vi "TRACTION WRITE FGV.vi"(7 "Enum - Menu":T1, 8 "error in (no error)":errorcluster, 11 "main ref":T2) -> (0 "error out":errorcluster)   [LabVIEW 2025]
uses:
  controls/LAB-IQ UI Data.ctl
  Traction Receipe Enum.ctl
  Traction Write enum.ctl
  d526d67c-090a-4194-9932-463c49b325c5.vi
panel:
  out "connection ID":refnum<k16>
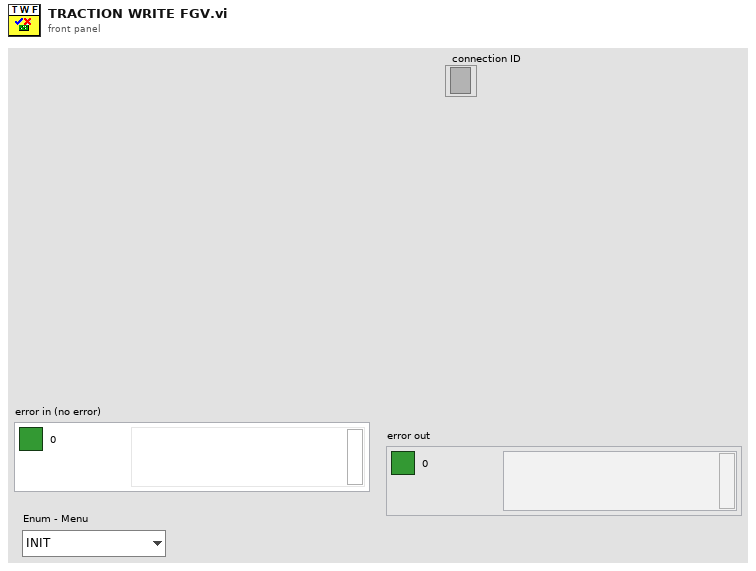
[diagram p1: front panel]
types:
  T1 = typedef "Traction Write enum.ctl" = enum16{"INIT", "WRITE", "CLOSE", "REINIT"}
  T2 = typedef "LAB-IQ UI Data.ctl" = cluster{"Main Home Screen":cluster{"GUI":refnum<vi>, "Platform Settings":refnum<vi>, "Configure":refnum<vi>, "Home":refnum<vi>, "EXIT":refnum<vi>, "service 2":refnum<vi>, "MainPage":refnum<vi>, "Analysis":refnum<vi>}, "Platform Settings":cluster{"mm/s  Surge":refnum<vi>, "Update Surge Speed":refnum<vi>, "Drive Error":refnum<vi>, "Disable Axis Jog Soft Limits":refnum<vi>, "mm/s  Sway":refnum<vi>, "Sway and Surge COM Status":refnum<vi>, "Heave COM Status":refnum<vi>, "Enable Platform":refnum<vi>, "Surge Forward Main":refnum<vi>, "Sway Right Main":refnum<vi>, "Sway Left Main":refnum<vi>, "Heave Down Main":refnum<vi>, "Heave Up main":refnum<vi>, "Update Sway Speed":refnum<vi>, "Update Heave Speed":refnum<vi>, "mm/s Heave":refnum<vi>, "mm/sec":refnum<vi>, "mm":refnum<vi>, "Surge Backward Main":refnum<vi>}, "Analysis Screen":cluster{"Analysis Home":refnum<vi>, "Surface Analysis":refnum<vi>, "Imaging":refnum<vi>, "Image Analysis":refnum<vi>, "Post Analysis":refnum<vi>}, "Config Screen":cluster{"Select Load Head":refnum<vi>, "Notes :":refnum<vi>, "FILE":refnum<vi>, "Sample ID :":refnum<vi>, "Operator ID :":refnum<vi>, "Operator Name :":refnum<vi>, "Auto":refnum<vi>}, "Motion Module":cluster{"zNL":refnum<vi>, "NL disp":refnum<vi>, "Rotary Tab":refnum<vi>, "Motion Direction:  3":refnum<vi>, "E.Velocity 2":refnum<vi>, "e.v/ssr 2":refnum<vi>, "Enter Fixed E.Velocity 2":refnum<vi>, "Enter Final SRR 2":refnum<vi>, "Enter initial SRR 2":refnum<vi>, "Enter Fixed SRR 2":refnum<vi>, "Enter the Final E.Velocity (m/s) 2":refnum<vi>, "Enter initial E.Velocity (m/s) 2":refnum<vi>, "Final Speed (RPM) 3":refnum<vi>, "Initial Speed (RPM) 2":refnum<vi>, "Enter the Final Velocity (m/s) 3":refnum<vi>, "Enter initial Velocity (m/s)  3":refnum<vi>, "Ramp Up 2":refnum<vi>, "TEST SELECTION":refnum<vi>, "SPEED SELECTION : ":refnum<vi>, "Angular Oscillation Set":refnum<vi>, "Traction":refnum<vi>, "Step Speed":refnum<vi>, "StepTable For Load-Speed":refnum<vi>, "StepTable For Speed":refnum<vi>, "Surge Forward MM":refnum<vi>, "Surge Backward MM":refnum<vi>, "M3 Image":refnum<vi>, "String 39":refnum<vi>, "Sway Left MM":refnum<vi>, "Sway Right MM":refnum<vi>, "Disable Axis Jog Soft Limits":refnum<vi>, "mm":refnum<vi>, "Heave Down MM":refnum<vi>, "Heave Up MM":refnum<vi>, "Wear Track Diameter (mm)":refnum<vi>, "Set WTD":refnum<vi>, "HomeScratch":refnum<vi>, "HomeRot":refnum<vi>, "PlaceModule":refnum<vi>, "Enter the Angle (Deg)":refnum<vi>, "Enter the Frequency (Hz)":refnum<vi>, "Motion Mode:":refnum<vi>, "LR Sway":refnum<vi>, "Rot Hor":refnum<vi>, "Scratch":refnum<vi>, "LR Cam":refnum<vi>, "MMBack":refnum<vi>, "MMNext":refnum<vi>, "Rot Ver":refnum<vi>, "Rotary Module Selection":refnum<vi>, "calculate rotary":refnum<vi>, "SPEED SELECTION : rotary":refnum<vi>, "Import 2":refnum<vi>, "Save 2":refnum<vi>, "File Path :  2":refnum<vi>, "String 45":refnum<vi>, "StepTable For Speed 3":refnum<vi>, "Enter the Speed(mm/sec)":refnum<vi>, "Enter the Speed(RPM)":refnum<vi>, "Enter Scratch Speed (mm/s):":refnum<vi>, "SwaySpeed Set":refnum<vi>, "Scartch Offset":refnum<vi>, "Motion type:":refnum<vi>, "HomeScratch 2":refnum<vi>, "Enter Scratch length (mm):":refnum<vi>, "Wear Track Diameter":refnum<vi>, "Rotary Speed Exced":refnum<vi>, "Scratch Mode":refnum<vi>, "No of Scratch":refnum<vi>}, "Environmental control":cluster{"Humidity  Status  3":refnum<vi>, "Low Temp  Status  2":refnum<vi>, "TK4 status 2":refnum<vi>, "Stage Temperature":refnum<vi>, "Sample Temperature":refnum<vi>, "Humidity (Amb)":refnum<vi>, "Clear List":refnum<vi>, "Add to list":refnum<vi>, "Wear":refnum<vi>, "Vibration":refnum<vi>, "Humidity (Chamber)":refnum<vi>, "Temperature (Chamber)":refnum<vi>, "ECR ":refnum<vi>, "Temperature (Amb)":refnum<vi>, "Microphone":refnum<vi>, "Acoustic Emission 3":refnum<vi>, "SNext":refnum<vi>, "APBack":refnum<vi>, "Enter the Temperature (°C):":refnum<vi>, "Enter the Stage \nTemperature (°C):":refnum<vi>, "Enter the Humidity (%Rh):":refnum<vi>, "Low Temp":refnum<vi>, "High Temp":refnum<vi>, "Humidity":refnum<vi>, "Sensors Picked":refnum<vi>}, "About Screen":cluster{"Password":refnum<vi>, "Home Service":refnum<vi>, "Advanced Setting":refnum<vi>, "About Tab":refnum<vi>, "ECR Port:":refnum<vi>, "Ramp Port:":refnum<vi>, "Installation/Replacement completed":refnum<vi>, "Loahead":refnum<vi>, "Heave and Surge COM Port:":refnum<vi>, "Sway COM Port:":refnum<vi>, "Temp Modbus:":refnum<vi>, "Humidity Port:":refnum<vi>, "Edit Gain Constants":refnum<vi>, "Save Gain Constants":refnum<vi>}, "Main Screen":cluster{"Main Screen Tab":refnum<vi>, "Angle and Frequency":refnum<vi>, "Stroke (mm)":refnum<vi>, "Angle (Deg)":refnum<vi>, "Main Speed Tab":refnum<vi>, "MTM MOTOR DISPLAY":refnum<vi>, "Disc Speed (m/sec)":refnum<vi>, "Ball Speed (m/sec)":refnum<vi>, "Disc Speed (RPM)":refnum<vi>, "Ball Speed (RPM)":refnum<vi>, "SPEED TAB":refnum<vi>, "Speed (m/sec)":refnum<vi>, "Set Speed (m/sec)":refnum<vi>, "Speed (RPM)":refnum<vi>, "Set Speed":refnum<vi>, "Time Tab":refnum<vi>, "Time ( HH:MM:SS ) 2":refnum<vi>, "Test Duration":refnum<vi>, "Test Duration 4":refnum<vi>, "TEST CYCLE":refnum<vi>, "TOTAL CYCLES":refnum<vi>, "Set Load (N)":refnum<vi>, "Temp Tabs":refnum<vi>, "Heater":refnum<vi>, "TK4 status":refnum<vi>, "ChamberTemp":refnum<vi>, "SetTmp":refnum<vi>, "Controller  Status":refnum<vi>, "ChamberTemp 2":refnum<vi>, "SetTmp 2":refnum<vi>, "Controller  Status 2":refnum<vi>, "ChamberTemp 3":refnum<vi>, "SetTmp 3":refnum<vi>, "Cooling":refnum<vi>, "Load Communication":refnum<vi>, "Ambient \nTemperature":refnum<vi>, "HumCOMStatus":refnum<vi>, "Ambient\n Humidity":refnum<vi>, "Freq (Hz)":refnum<vi>, "Load En":refnum<vi>, "NLt":refnum<vi>, "zNL 2":refnum<vi>, "Humidity On":refnum<vi>, "humidity disp":refnum<vi>, "Set Humidity":refnum<vi>, "NL disp 2":refnum<vi>, "Humidity On 2":refnum<vi>, "humidity disp 2":refnum<vi>, "Set Humidity 2":refnum<vi>, "NL disp 3":refnum<vi>, "AppLoadSeq scratch":refnum<vi>, "Stop Scratch":refnum<vi>, "ClrLog":refnum<vi>, "Trip Log":refnum<vi>, "STOP":refnum<vi>, "Start Test":refnum<vi>, "Test status":refnum<vi>, "AR Led":refnum<vi>, "Data":refnum<vi>, "Health":refnum<vi>, "Sway COM Status":refnum<vi>, "Heave COM Status":refnum<vi>, "Grp Tab":refnum<vi>, "Sub Graph":refnum<vi>, "SD (mm)":refnum<vi>, "Siliding distance Reset Graph":refnum<vi>, "SDGp":refnum<vi>, "Humidity Reset Graph":refnum<vi>, "HumrGp":refnum<vi>, "Acoustic Emission (mV)":refnum<vi>, "Aqucostic Reset Graph":refnum<vi>, "gACQUOS":refnum<vi>, "ECR RESET":refnum<vi>, "ECR":refnum<vi>, "Temperature Reset":refnum<vi>, "Acoustic Emission (mV) 2":refnum<vi>, "Aqucostic Reset Graph 2":refnum<vi>, "gACQUOS 2":refnum<vi>, "ECR RESET 2":refnum<vi>, "ECR 2":refnum<vi>, "Temperature Reset 2":refnum<vi>, "Temperature (deg c)":refnum<vi>, "Speed Reset Graph":refnum<vi>, "Speed Tab":refnum<vi>, "MTM DISC  SPEED":refnum<vi>, "MTM BALL SPEED":refnum<vi>, "speed mm/sec":refnum<vi>, "Hymidity":refnum<vi>, "Humidity Disable trip":refnum<vi>, "CoF Trip  2":refnum<vi>, "Depth Trip":refnum<vi>, "Weart Deapth":refnum<vi>, "Depth Reset Graph":refnum<vi>, "Weart":refnum<vi>, "Depthz":refnum<vi>, "Depth (µm)":refnum<vi>, "WearGp":refnum<vi>, "NL Trip 2":refnum<vi>, "Load pid":refnum<vi>, "Load Disable Trip":refnum<vi>, "Load Reset Graph":refnum<vi>, "NL Display 4":refnum<vi>, "Main Chart 3":refnum<vi>, "BACK":refnum<vi>, "Depth Trip 2":refnum<vi>, "COF TRIP ":refnum<vi>, "Friction Force (N)":refnum<vi>, "FF Reset Graph":refnum<vi>, "FF Disable Trip":refnum<vi>, "FF TRIP":refnum<vi>, "COF Disable Trip":refnum<vi>, "COF Reset Graph":refnum<vi>, "Start Test Temp":refnum<vi>, "zFF":refnum<vi>, "Friction Force (N) Graph":refnum<vi>, "Coefficient of Friction":refnum<vi>, "Scratch Start Test":refnum<vi>, "FF Tab":refnum<vi>, "Cyclic Friction Force (N)":refnum<vi>, "CZ FF":refnum<vi>, "Cyclic Friction Force (N) Graph":refnum<vi>, "Cyclic Coefficient of Friction":refnum<vi>, "Cyclic FF TRIP":refnum<vi>, "Cyclic FF Disable Trip":refnum<vi>, "cyclic COF Disable Trip":refnum<vi>, "cyclic COF TRIP":refnum<vi>, "cyclic COF Reset Graph":refnum<vi>, "Cyclic FF Reset Graph":refnum<vi>, "Test Trip":refnum<vi>, "Multi Scratch Pass":refnum<vi>, "Scratch Start Recording":refnum<vi>}, "Loading":cluster{"Indentation":refnum<vi>, "Reference Sample":refnum<vi>, "Load Cell Communication Slide":refnum<vi>, "com 3":refnum<vi>, "com":refnum<vi>, "DecaForce COM Status":refnum<vi>, "Update":refnum<vi>, "Clear 3":refnum<vi>, "seq":refnum<vi>, "Stribeck table":refnum<vi>, "Stribeck Table  For loading":refnum<vi>, "Loading Mode":refnum<vi>, "Enter the Final Load (N)":refnum<vi>, "Enter the CoF Trip":refnum<vi>, "Enter the Friction Force Trip":refnum<vi>, "Enter the Normal load Trip":refnum<vi>, "Enter the Load  (N)":refnum<vi>, "KiloForce":refnum<vi>, "DecaForce ":refnum<vi>, "MicroForce":refnum<vi>, "LHBack":refnum<vi>, "LHNext":refnum<vi>, "Enter the Loading Rate (N/min)":refnum<vi>, "Message":refnum<vi>, "Warning 2":refnum<vi>, "SSP 0.75":refnum<vi>, "SSP 0.5":refnum<vi>, "SSP 0.3":refnum<vi>, "Warning":refnum<vi>, "gui GIF":refnum<vi>, "Communication is established":refnum<vi>, "AppLoad 4":refnum<vi>, "Multipoint":refnum<vi>, "Load Selection":refnum<vi>}, "PID":cluster{"Ramp MulFac":refnum<vi>, "pulses LoadDiffRamp(2..10)":refnum<vi>, "PulseControlRamp(diff<=3N)":refnum<vi>, "SetLoadDeadband(%) Load(0-10N)":refnum<vi>, "PID gains out delay (microForce)":refnum<vi>, "Ramp":refnum<vi>, "Gain 2":refnum<vi>, "pulses LoadDiff(2..10)":refnum<vi>, "pulses LoadDiff(11..50)":refnum<vi>, "PulseControl(diff<=3N)":refnum<vi>, "SetLoadDeadband(%)  2":refnum<vi>, "Dummy Run":refnum<vi>, "Vertical load (N)":refnum<vi>, "AutoTune":refnum<vi>, "Offset 3 ":refnum<vi>, "apply load":refnum<vi>, "Offset  3":refnum<vi>, "apply load 2":refnum<vi>, "Enter ByPass Load":refnum<vi>, "reinit 3":refnum<vi>, "output range delay":refnum<vi>, "PID gains out delay":refnum<vi>, "Bypass Load":refnum<vi>, "pulsesSent":refnum<vi>, "pulses ":refnum<vi>, "actpid":refnum<vi>, "gFF Rot":refnum<vi>, "pulses LoadDiff(21..1000)":refnum<vi>, "Delay":refnum<vi>, "deadband":refnum<vi>}, "Config Parameters":cluster{"Tab Control 3":refnum<vi>, "Tab Control 19":refnum<vi>, "SAMPLES":refnum<vi>, "Re-initilaize":refnum<vi>, "Filter ON/OFF":refnum<vi>, "TracHomeSurgeOffsetCounts 10MM":refnum<vi>, "TracHomeSwayOffsetCounts 10MM":refnum<vi>, "Acoustic Emission:":refnum<vi>, "Apply Filter (FF)":refnum<vi>, "Filter% 2":refnum<vi>, "Apply Filter (Load)":refnum<vi>, "Filter% ":refnum<vi>, "Sway distance (mm)":refnum<vi>, "Surge distance (mm)":refnum<vi>, "DataSavingLoopDelay(ms)":refnum<vi>, "SAVE 2":refnum<vi>, "Enter Distance":refnum<vi>, "Sway Counts:":refnum<vi>, "Distance (mm): 3":refnum<vi>, "Surge Counts:":refnum<vi>, "Distance (mm): 2":refnum<vi>, "Distance (mm):":refnum<vi>, "Heave Counts:":refnum<vi>, "LRMHomeSurgeOffsetCounts":refnum<vi>, "LRMHomeSwayOffsetCounts":refnum<vi>, "TracHomeSurgeOffsetCounts 20MM":refnum<vi>, "TracHomeSwayOffsetCounts 20MM":refnum<vi>, "RotHomeSwayOffsetCounts":refnum<vi>, "RotHomeSurgeOffsetCounts":refnum<vi>, "Heave distance":refnum<vi>, "Zmm":refnum<vi>, "Heave Pulses/mm":refnum<vi>, "Surge Pulses/mm":refnum<vi>, "Sway Pulses/mm":refnum<vi>, "Heave Pitch":refnum<vi>, "Surge Pitch":refnum<vi>, "Sway Pitch":refnum<vi>, "Heave PPR":refnum<vi>, "Surge PPR":refnum<vi>, "Sway PPR":refnum<vi>, "Tab Control 5":refnum<vi>, "Tab Control 14":refnum<vi>, "Tab Control 26":refnum<vi>, "AE":refnum<vi>, "Heave Loop Delay":refnum<vi>, "Heave PID Speed":refnum<vi>, "Surge Jog Speed":refnum<vi>, "Heave Jog Speed":refnum<vi>, "Sway Loop Delay":refnum<vi>, "Sway PID Speed":refnum<vi>, "Sway Jog Speed":refnum<vi>, "DEPTH TRIP VALUE":refnum<vi>, "LOAD TRIP VALUE":refnum<vi>, "DEPTH TRIP   ENABLE":refnum<vi>, "LOAD TRIP  ENABLE":refnum<vi>, "CYCLIC FF TRIP VALUE":refnum<vi>, "FF TRIP VALUE":refnum<vi>, "CYCLIC CoF TRIP VALUE":refnum<vi>, "COF TRIP VALUE":refnum<vi>, "CYCLIC COF TRIP  ENABLE":refnum<vi>, "CYCLIC FF TRIP  ENABLE":refnum<vi>, "FF TRIP  ENABLE":refnum<vi>, "COF TRIP  ENABLE":refnum<vi>, "JOG TRIP LOAD VALUE (N)":refnum<vi>}, "Loading Com Port":cluster{"ClearAll":refnum<vi>, "Mz(Nm)":refnum<vi>, "My(Nm)":refnum<vi>, "Mx(Nm)":refnum<vi>, "Save Dwell":refnum<vi>, "Mx ":refnum<vi>, "My ":refnum<vi>, "Mz":refnum<vi>, "Fx(N)":refnum<vi>, "Fy(N)":refnum<vi>, "Fz(N)":refnum<vi>, "ZeroAll":refnum<vi>, "Acq Delay (ms)":refnum<vi>, "Burst Delay (ms)":refnum<vi>, "model":refnum<vi>, "SN":refnum<vi>, "FFx(N)":refnum<vi>, "Sensor IP":refnum<vi>, "Port":refnum<vi>, "FFy(N)":refnum<vi>, "Load(N)":refnum<vi>, "delete Handle":refnum<vi>, "Create Handle":refnum<vi>, "ft_data":refnum<vi>, "ft_range":refnum<vi>, "ft_data 2":refnum<vi>, "stop 6":refnum<vi>, "running_flag":refnum<vi>, "ft_udp_handle":refnum<vi>, "get-data-return":refnum<vi>, "get-range-return":refnum<vi>, "zero-return":refnum<vi>, "filter-return":refnum<vi>, "initial-return":refnum<vi>, "deleteHandle-result":refnum<vi>, "Load Cell Temp":refnum<vi>}, "Heave AND Surge":cluster{"SURGE POSE":refnum<vi>, "error out Read":refnum<vi>, "HEAVE POSE":refnum<vi>, "State":refnum<vi>, "Homed":refnum<vi>, "Sequence ID":refnum<vi>, "error out Write":refnum<vi>, "faultCode":refnum<vi>, "Ack ID":refnum<vi>, "SPEED":refnum<vi>, "Distance":refnum<vi>, "Mode Command":refnum<vi>, "Heave and Surge Read":refnum<vi>, "Read Heave Temp":refnum<vi>, "Spare 15":refnum<vi>, "Spare 14":refnum<vi>, "Spare 13":refnum<vi>, "Spare 12":refnum<vi>, "Spare 11":refnum<vi>, "Spare 10":refnum<vi>, "Spare 9":refnum<vi>, "Spare 8":refnum<vi>, "Spare 7":refnum<vi>, "Spare 6":refnum<vi>, "Spare 5":refnum<vi>, "Spare 4":refnum<vi>, "Spare 2":refnum<vi>, "Spare 1":refnum<vi>, "Node Id":refnum<vi>, "Spare 3":refnum<vi>, "SPARE 4":refnum<vi>, "SPARE 3":refnum<vi>, "SPARE 2":refnum<vi>, "SPARE 1":refnum<vi>, "fwMajor":refnum<vi>, "fwMinor":refnum<vi>, "Manual Write":refnum<vi>, "Heave and Surge Write":refnum<vi>, "SPARE 5":refnum<vi>, "Reserved ":refnum<vi>, "SPARE 8":refnum<vi>, "SPARE 6":refnum<vi>, "SPARE 7":refnum<vi>, "SPARE 17":refnum<vi>, "SPARE 16":refnum<vi>, "SPARE 15":refnum<vi>, "SPARE 14":refnum<vi>, "SPARE 13":refnum<vi>, "SPARE 12":refnum<vi>, "SPARE 11":refnum<vi>, "SPARE 10":refnum<vi>, "SPARE 9":refnum<vi>, "System UPTIME":refnum<vi>, "Missed Packets":refnum<vi>, "faultCode Surge Right":refnum<vi>, "faultCode Surge Left":refnum<vi>, "faultCode Heave":refnum<vi>}, "New PID LOGIC":cluster{"Fine Tune Zone":refnum<vi>, "PID SDelay":refnum<vi>, "Max_pos_limit":refnum<vi>, "Min_pos_limit":refnum<vi>, "i_limit":refnum<vi>, "pct_scale":refnum<vi>, "Deadband":refnum<vi>, "Kd":refnum<vi>, "Ki":refnum<vi>, "Kp":refnum<vi>, "Current Position":refnum<vi>, "Set Load":refnum<vi>, "Current Load":refnum<vi>, "Pulse delta":refnum<vi>, "Init Step":refnum<vi>, "Max Step Linit":refnum<vi>, "min_deadband_floor":refnum<vi>, "dynamic_spindle_noise_scalar":refnum<vi>, "min_finetune_floor":refnum<vi>, "filter_alpha":refnum<vi>}, "SWAY ":cluster{"fwMajor":refnum<vi>, "Homed":refnum<vi>, "Rotary POSE":refnum<vi>, "State":refnum<vi>, "SWAY POSE":refnum<vi>, "Ack ID":refnum<vi>, "faultCode":refnum<vi>, "Node Id":refnum<vi>, "fwMinor":refnum<vi>, "Spare 6":refnum<vi>, "Spare 5":refnum<vi>, "Spare 4":refnum<vi>, "Spare 3":refnum<vi>, "Spare 2":refnum<vi>, "Spare 1":refnum<vi>, "Spare 7":refnum<vi>, "SPARE  5":refnum<vi>, "error out Write  SWAY ":refnum<vi>, "error out Read SWAY ":refnum<vi>, "Manual Write SWAY ":refnum<vi>, "SWAY WRITE":refnum<vi>, "SPARE  4":refnum<vi>, "SPARE  3":refnum<vi>, "SPARE 2":refnum<vi>, "SPARE 1":refnum<vi>, "Spare 15":refnum<vi>, "Spare 14":refnum<vi>, "Spare 13":refnum<vi>, "Spare 12":refnum<vi>, "Spare 11":refnum<vi>, "Spare 9":refnum<vi>, "Spare 8":refnum<vi>, "SPEED":refnum<vi>, "Distance":refnum<vi>, "Mode Command":refnum<vi>, "Sequence ID":refnum<vi>, "SWAY READ":refnum<vi>, "Spare 10":refnum<vi>, "Read SWAY Temp":refnum<vi>, "faultCode Sway ":refnum<vi>, "Missed Packets":refnum<vi>, "System UPTIME sway":refnum<vi>, "SPARE 6":refnum<vi>, "SPARE 7":refnum<vi>, "SPARE 9":refnum<vi>, "SPARE 11":refnum<vi>, "SPARE 10":refnum<vi>, "SPARE 8":refnum<vi>, "SPARE 13":refnum<vi>, "SPARE 12":refnum<vi>, "SPARE 17":refnum<vi>, "SPARE 16":refnum<vi>, "SPARE 15":refnum<vi>, "SPARE 14":refnum<vi>, "Reserved":refnum<vi>, "faultCode Rotary":refnum<vi>}, "Analysis Screen":cluster{"Analysis Home":refnum<vi>, "Refresh 2":refnum<vi>, "MEAN 4":refnum<vi>, "SD 4":refnum<vi>, "VARIANCE 4":refnum<vi>, "MEAN  3":refnum<vi>, "SD  3":refnum<vi>, "VARIANCE  3":refnum<vi>, "MEAN 2":refnum<vi>, "SD  2":refnum<vi>, "VARIANCE 2":refnum<vi>, "MEAN":refnum<vi>, "SD":refnum<vi>, "VARIANCE":refnum<vi>, "File 4 Discription":refnum<vi>, "OPEN 4":refnum<vi>, "File Name 4":refnum<vi>, "OPEN 3":refnum<vi>, "File 3 Discription":refnum<vi>, "File Name 3":refnum<vi>, "Y-AXIS":refnum<vi>, "X-AXIS":refnum<vi>, "XY Graph":refnum<vi>, "File Name 2":refnum<vi>, "File Name 1":refnum<vi>, "OPEN 2":refnum<vi>, "OPEN 1":refnum<vi>, "File 1 Discription ":refnum<vi>, "File 2 Discription":refnum<vi>, "Export":refnum<vi>, "File Format":refnum<vi>}, "Traction":cluster{"faultCode Traction 2":refnum<vi>, "faultCode Traction 1":refnum<vi>, "Missed Packets":refnum<vi>, "System UPTIME Traction":refnum<vi>, "SPARE 17":refnum<vi>, "SPARE 16":refnum<vi>, "SPARE 15":refnum<vi>, "SPARE 14":refnum<vi>, "SPARE 13":refnum<vi>, "SPARE 12":refnum<vi>, "SPARE 11":refnum<vi>, "SPARE 10":refnum<vi>, "SPARE 9":refnum<vi>, "SPARE 8":refnum<vi>, "SPARE 7":refnum<vi>, "SPARE 6":refnum<vi>, "Reserved":refnum<vi>, "SPARE  5":refnum<vi>, "Manual Write TRACTION":refnum<vi>, "TRACTION WRITE":refnum<vi>, "SPARE  4":refnum<vi>, "SPARE  3":refnum<vi>, "SPARE 2":refnum<vi>, "SPARE 1":refnum<vi>, "Spare 7":refnum<vi>, "Spare 6":refnum<vi>, "Spare 5":refnum<vi>, "Spare 4":refnum<vi>, "Spare 2":refnum<vi>, "Spare 1":refnum<vi>, "Node Id":refnum<vi>, "Read TRACTION Temp":refnum<vi>, "fwMinor":refnum<vi>, "fwMajor":refnum<vi>, "faultCode":refnum<vi>, "TRACTION POSE":refnum<vi>, "TRACTION POSE 2":refnum<vi>, "Homed":refnum<vi>, "State":refnum<vi>, "Ack ID":refnum<vi>, "SPEED":refnum<vi>, "Distance":refnum<vi>, "Mode Command":refnum<vi>, "Sequence ID":refnum<vi>, "error out Read TRACTION":refnum<vi>, "error out Write  TRACTION":refnum<vi>, "TRACTION READ":refnum<vi>, "Spare 3":refnum<vi>}, "Traction reciepe":cluster{"SRR Sweep Range (%) Stribeck":refnum<vi>, "Traction Receipe":refnum<vi>, "Total Execution Time":refnum<vi>, "Total Steps":refnum<vi>, "Duration / Step (s)  Stribeck":refnum<vi>, "STRIBECK Fixed SRR List (%)":refnum<vi>, "Duration / Step (s) Traction":refnum<vi>, "SRR Sweep Range (%) traction":refnum<vi>, "Rolling Speed (mm/s)":refnum<vi>, "Temperature Stages (°C)":refnum<vi>, "Ball Load (N)":refnum<vi>, "Lubricant Name":refnum<vi>, "Profile File Name":refnum<vi>, "SET entrainment Velocity":refnum<vi>, "Test Array Size":refnum<vi>, "SRR INDEX [ STRIBECK]":refnum<vi>, "Stribeck Size":refnum<vi>, "SET SRR":refnum<vi>, "ELAPSED TIMER ":refnum<vi>, "BALL SET RPM":refnum<vi>, "DISC SET RPM":refnum<vi>, "SET LOAD":refnum<vi>, "TEMPERATURE READ":refnum<vi>, "SET TEMPERATURE":refnum<vi>, "Traction Size":refnum<vi>, "DISC SPEED (rpm)":refnum<vi>, "BALL SPEED (rpm)":refnum<vi>, "BALL WEAR TRACK":refnum<vi>, "DISC WEARTRACK":refnum<vi>, "SRR INDEX [ TRACTION]":refnum<vi>, "Start Index Type":refnum<vi>, "Enum - Menu":refnum<vi>, "Ball (mm/sec)":refnum<vi>, "Disc (mm/sec)":refnum<vi>}, "Traction Control":cluster{"HomeTraction":refnum<vi>, "Demo Mode Display":refnum<vi>, "Traction Message":refnum<vi>, "Traction Step Update Details":refnum<vi>, "Main Tab sequence for selection":refnum<vi>, "Ramp Tab":refnum<vi>, "e.v/ssr":refnum<vi>, "Enter Fixed E.Velocity":refnum<vi>, "Enter Final SRR":refnum<vi>, "Enter initial SRR":refnum<vi>, "Enter Fixed SRR":refnum<vi>, "Enter the Final E.Velocity (m/s)":refnum<vi>, "Enter initial E.Velocity (m/s)":refnum<vi>, "Ball WTD":refnum<vi>, "E.Velocity":refnum<vi>, "Enter the Final Velocity (m/s)":refnum<vi>, "Enter initial Velocity (m/s)":refnum<vi>, "Ramp Up   Disc":refnum<vi>, "Initial DiscSpeed (RPM)":refnum<vi>, "Final Speed (RPM) Ball":refnum<vi>, "Final Speed (RPM)":refnum<vi>, "Initial Speed (RPM) Ball":refnum<vi>, "Enter the Final Velocity (m/s) Ball":refnum<vi>, "Enter initial Velocity (m/s) Ball":refnum<vi>, "Ramp Up":refnum<vi>, "ExceedBallSpeed step":refnum<vi>, "ExceedDiscSpeed":refnum<vi>, "BallSpeed Exceed Indication":refnum<vi>, "Apply":refnum<vi>, "SPEED SELECTION : MTM":refnum<vi>, "SPEED SELECTION : MTM 2":refnum<vi>, "TEST SELECTION (MTM)":refnum<vi>, "MTM Test Selection":refnum<vi>, "File Path Tab":refnum<vi>, "File Path String":refnum<vi>, "Save":refnum<vi>, "Save  2":refnum<vi>, "Import ":refnum<vi>, "File Path :":refnum<vi>, "Step Sequence Indication Tab":refnum<vi>, "Step Sequence Indication":refnum<vi>, "Calculate Step":refnum<vi>, "StepTable":refnum<vi>, "ExceedDiscSpeed  Cinstant Speed":refnum<vi>, "ExceedBallSpeed Constant":refnum<vi>, "TEST SELECTION (MTM) 2":refnum<vi>, "SPEED SELECTION : MTM 3":refnum<vi>, "MTM Test Selection 2":refnum<vi>, "Enter the Speed (m/sec): ":refnum<vi>, "Enter the Speed (m/sec):  2":refnum<vi>, "Enter the Speed (RPM):":refnum<vi>, "Lower Spped ":refnum<vi>, "Upper":refnum<vi>, "Enter the Speed (RPM):Ball":refnum<vi>, "Disc Motion Direction: ":refnum<vi>, "Ball Motion Direction :":refnum<vi>, "Motion Mode: ":refnum<vi>, "Wear Track Diameter (mm) ":refnum<vi>, "Disc Speed Indicator":refnum<vi>, "ExceedBallSpeed":refnum<vi>}}
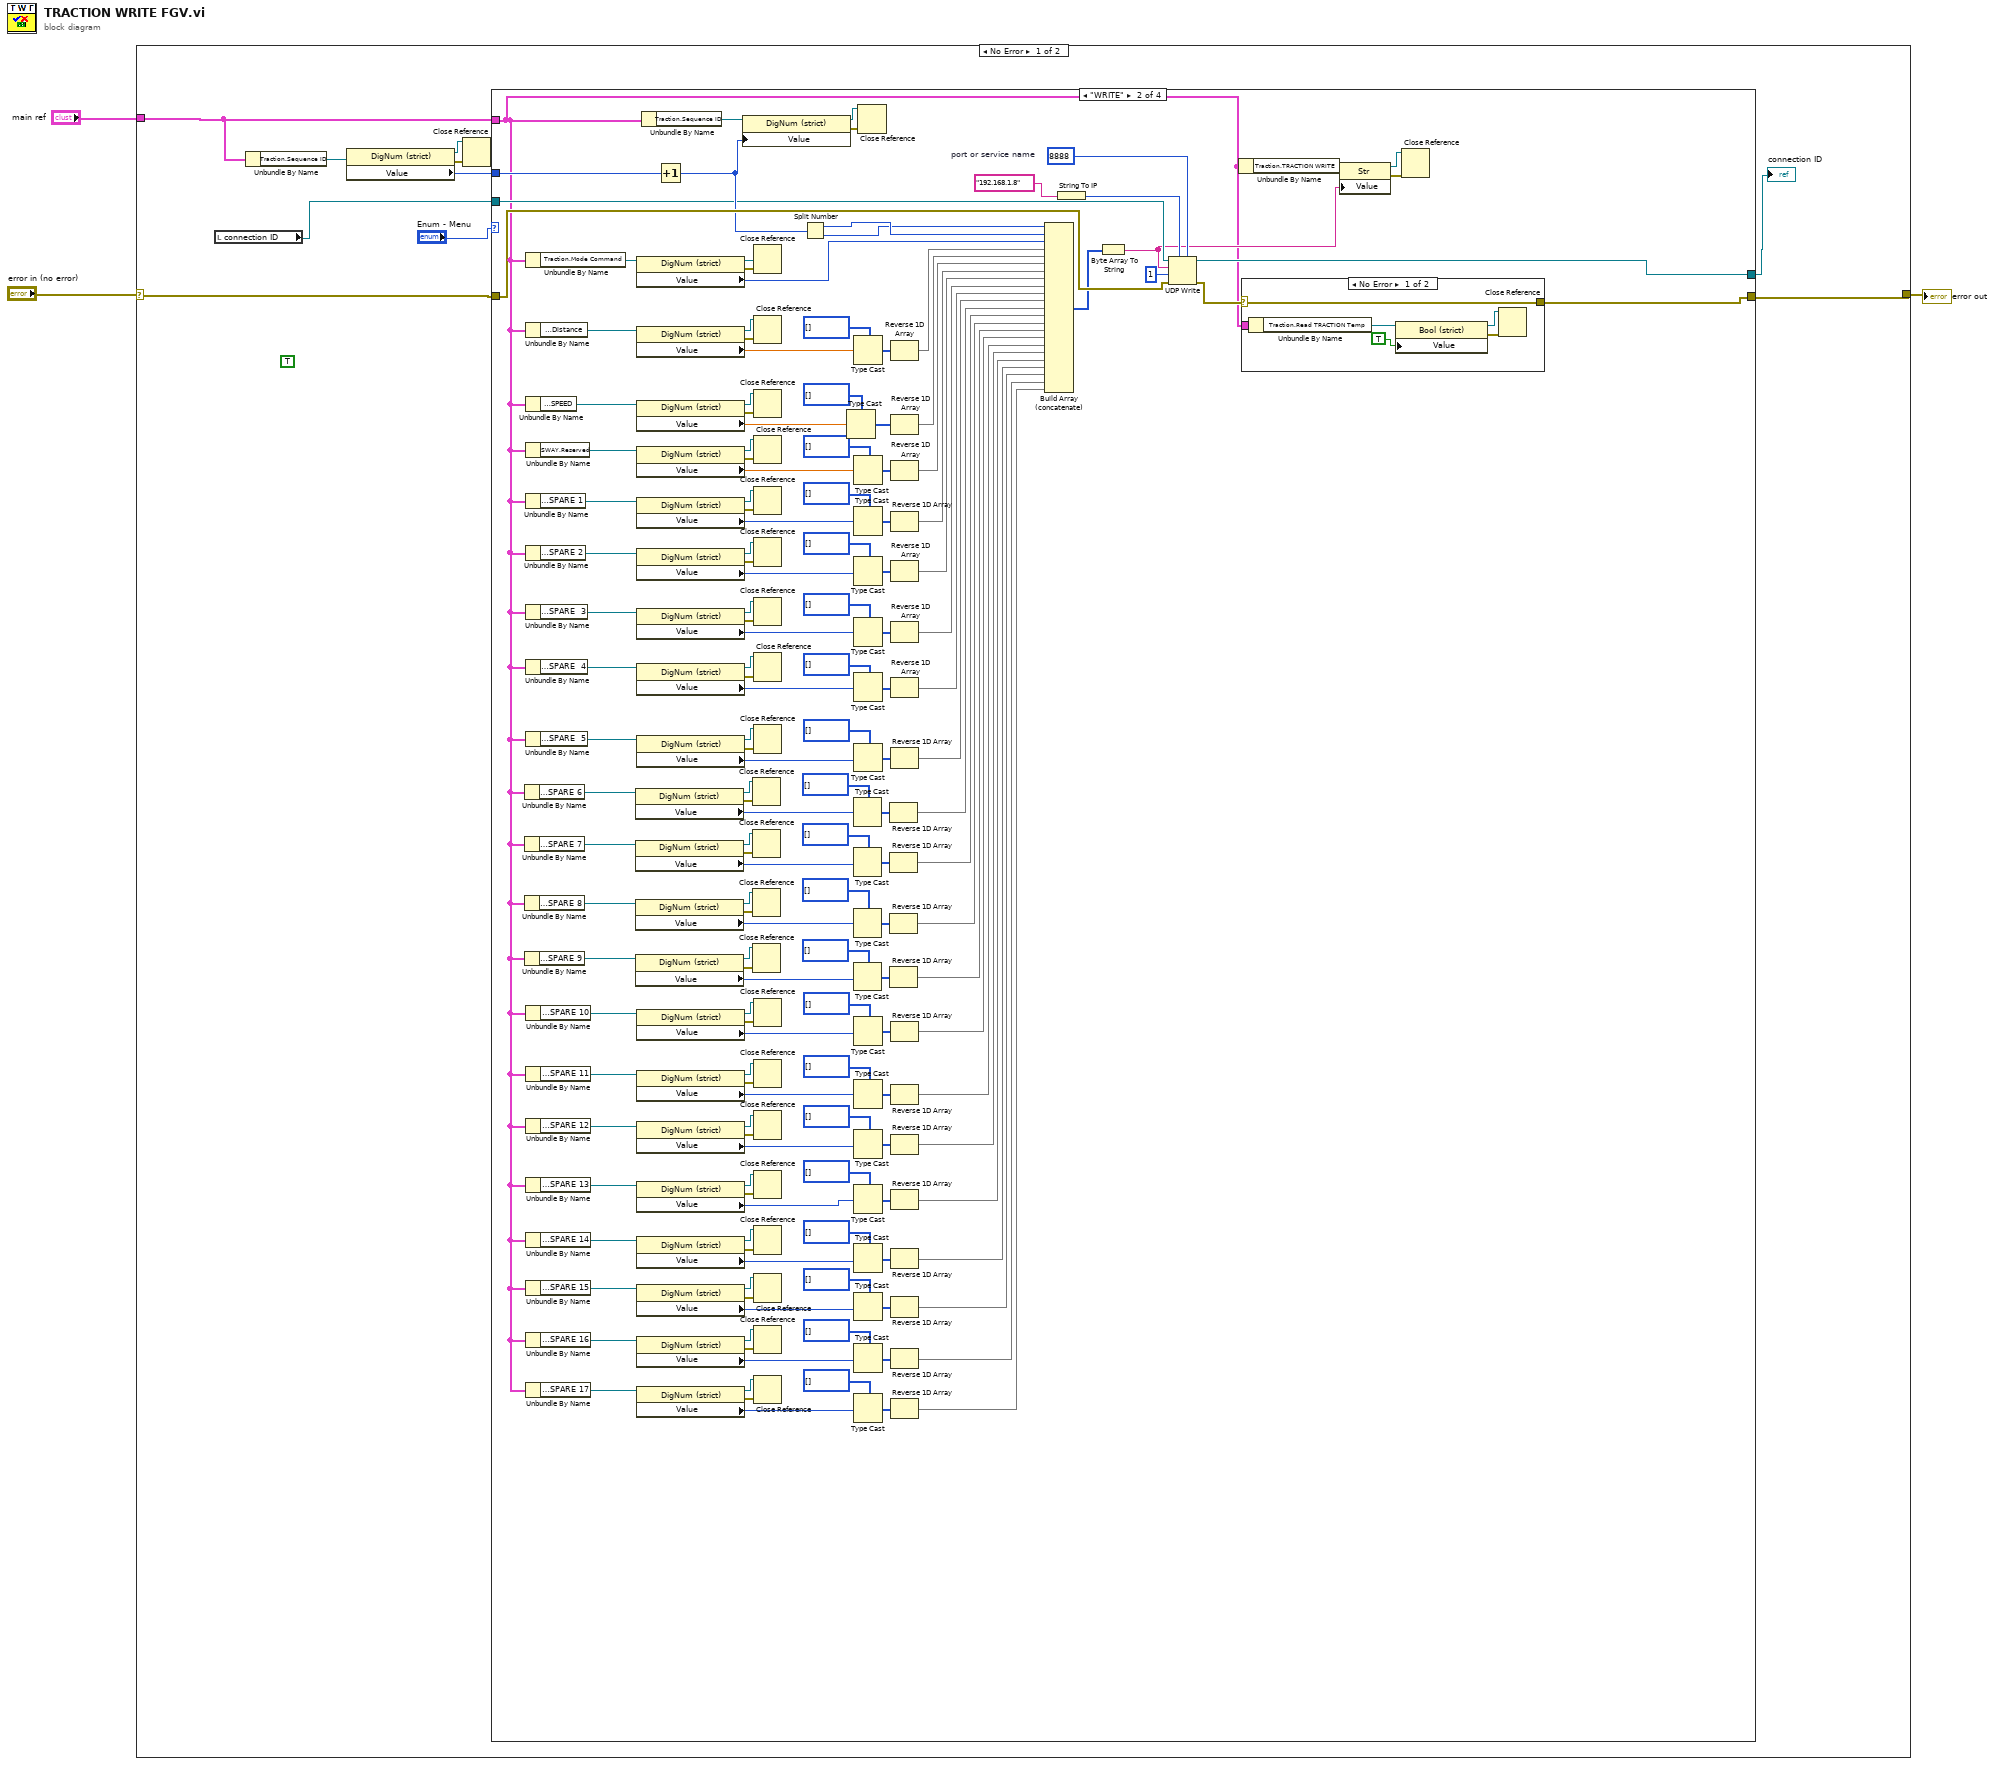
[diagram p0: block diagram]
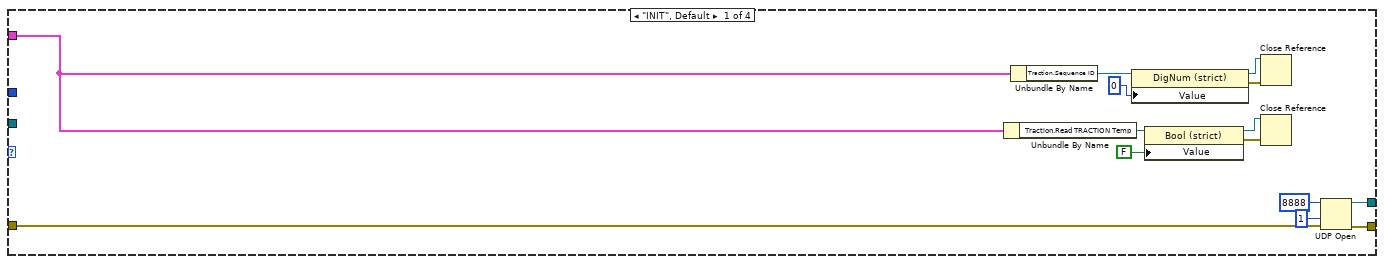
[diagram p2: hidden frame]
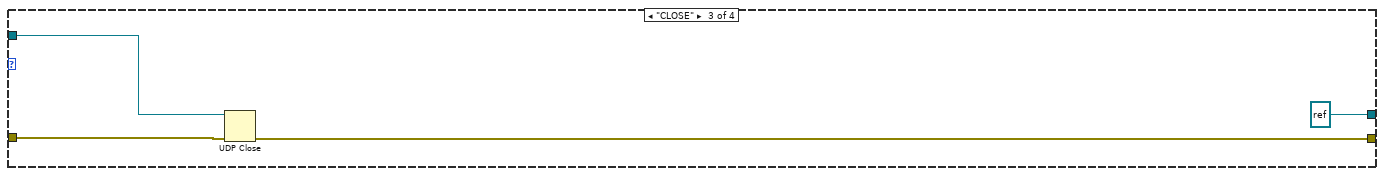
[diagram p4: hidden frame]
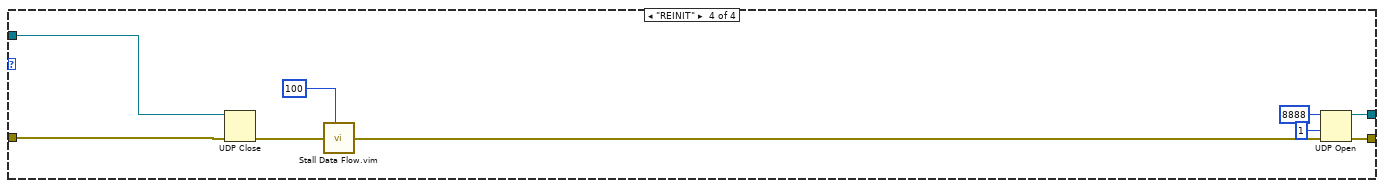
[diagram p5: hidden frame]
diagram:
  n1 = case shown="No Error" "error in (no error)" {
    selector: "error in (no error)" -> [w13 _]
    tunnel: "main ref" -> [w11 _]
    tunnel: [w12 _] -> w1
    frame No Error {
      (unwired) TRUE
      n2 = local read "connection ID"() -> (w5:refnum<k16>)
      n3 = Unbundle By Name(w11) -> ("Traction.Sequence ID"=w7:refnum<vi>)
      n4 = property class="DigNum (strict)"(reference=w7) -> (reference out=w9:refnum<vi>, error out=w8:errorcluster, "Value"=w6:u16)  [unwired: 1 in]
      n5 = Close Reference(reference=w9, error in (no error)=w8) -> ()  [unwired: 1 out]
      n6 = case shown="\"WRITE\"" "Enum - Menu" {
        tunnel: w13 -> [w26 w191 w203 w212]
        tunnel: [w25 w161 w201 w206] -> w12
        tunnel: [w24 w190 refnum<k16> refnum ("connection ID out") w205] -> w4
        tunnel: w11 -> [w15 w40 _ _]
        tunnel: w6 -> [_ w185 _ _]
        tunnel: w5 -> [_ w160 w202 w211]
        frame "INIT", Default {
          n7 = Unbundle By Name(w15) -> ("Traction.Read TRACTION Temp"=w19:refnum<vi>)
          n8 = Unbundle By Name(w15) -> ("Traction.Sequence ID"=w23:refnum<vi>)
          n9 = property class="DigNum (strict)"(reference=w23, "Value"=u16 0) -> (reference out=w21:refnum<vi>, error out=w22:errorcluster)  [unwired: 1 in]
          n10 = property class="Bool (strict)"(reference=w19, "Value"=FALSE) -> (reference out=w17:refnum<vi>, error out=w18:errorcluster)  [unwired: 1 in]
          n11 = Close Reference(reference=w21, error in (no error)=w22) -> ()  [unwired: 1 out]
          n12 = Close Reference(reference=w17, error in (no error)=w18) -> ()  [unwired: 1 out]
          n13 = UDP Open(8:w26, 9:1 ("timeout ms (25000)"), 11:u16 8888 ("port")) -> (port=w24:refnum<k16>, 0:w25:errorcluster)  [unwired: 2 in, 1 out]
        }
        frame "WRITE" {
          w193 = u16 8888  # port or service name
          n14 = Unbundle By Name(w40) -> ("Traction.SPARE 6"=w109:refnum<vi>)
          n15 = Unbundle By Name(w40) -> ("Traction.SPARE 7"=w106:refnum<vi>)
          n16 = Unbundle By Name(w40) -> ("Traction.SPARE 8"=w103:refnum<vi>)
          n17 = Unbundle By Name(w40) -> ("Traction.SPARE 9"=w100:refnum<vi>)
          n18 = Unbundle By Name(w40) -> ("Traction.Mode Command"=w180:refnum<vi>)
          n19 = Unbundle By Name(w40) -> ("Traction.Distance"=w176:refnum<vi>)
          n20 = Unbundle By Name(w40) -> ("Traction.SPEED"=w169:refnum<vi>)
          n21 = Unbundle By Name(w40) -> ("SWAY.Reserved"=w115:refnum<vi>)
          n22 = Unbundle By Name(w40) -> ("Traction.SPARE 1"=w156:refnum<vi>)
          n23 = Unbundle By Name(w40) -> ("Traction.SPARE 2"=w153:refnum<vi>)
          n24 = Unbundle By Name(w40) -> ("Traction.SPARE  3"=w150:refnum<vi>)
          n25 = Unbundle By Name(w40) -> ("Traction.SPARE  4"=w147:refnum<vi>)
          n26 = Unbundle By Name(w40) -> ("Traction.SPARE  5"=w127:refnum<vi>)
          n27 = Unbundle By Name(w40) -> ("Traction.SPARE 10"=w84:refnum<vi>)
          n28 = Unbundle By Name(w40) -> ("Traction.SPARE 11"=w79:refnum<vi>)
          n29 = Unbundle By Name(w40) -> ("Traction.SPARE 12"=w76:refnum<vi>)
          n30 = Unbundle By Name(w40) -> ("Traction.SPARE 13"=w73:refnum<vi>)
          n31 = Unbundle By Name(w40) -> ("Traction.SPARE 14"=w70:refnum<vi>)
          n32 = Unbundle By Name(w40) -> ("Traction.SPARE 15"=w54:refnum<vi>)
          n33 = Unbundle By Name(w40) -> ("Traction.SPARE 16"=w51:refnum<vi>)
          n34 = Unbundle By Name(w40) -> ("Traction.SPARE 17"=w42:refnum<vi>)
          n35 = property class="DigNum (strict)"(reference=w109) -> (reference out=w108:refnum<vi>, error out=w110:errorcluster, "Value"=w98:u8)  [unwired: 1 in]
          n36 = property class="DigNum (strict)"(reference=w106) -> (reference out=w107:refnum<vi>, error out=w105:errorcluster, "Value"=w95:u8)  [unwired: 1 in]
          n37 = property class="DigNum (strict)"(reference=w103) -> (reference out=w102:refnum<vi>, error out=w104:errorcluster, "Value"=w89:u8)  [unwired: 1 in]
          n38 = property class="DigNum (strict)"(reference=w100) -> (reference out=w101:refnum<vi>, error out=w99:errorcluster, "Value"=w90:u8)  [unwired: 1 in]
          n39 = property class="DigNum (strict)"(reference=w180) -> (reference out=w179:refnum<vi>, error out=w181:errorcluster, "Value"=w178:u8)  [unwired: 1 in]
          n40 = property class="DigNum (strict)"(reference=w176) -> (reference out=w177:refnum<vi>, error out=w175:errorcluster, "Value"=w174:sgl)  [unwired: 1 in]
          n41 = property class="DigNum (strict)"(reference=w169) -> (reference out=w170:refnum<vi>, error out=w168:errorcluster, "Value"=w165:sgl)  [unwired: 1 in]
          n42 = property class="DigNum (strict)"(reference=w115) -> (reference out=w114:refnum<vi>, error out=w116:errorcluster, "Value"=w119:sgl)  [unwired: 1 in]
          n43 = property class="DigNum (strict)"(reference=w156) -> (reference out=w155:refnum<vi>, error out=w157:errorcluster, "Value"=w145:u8)  [unwired: 1 in]
          n44 = property class="DigNum (strict)"(reference=w153) -> (reference out=w154:refnum<vi>, error out=w152:errorcluster, "Value"=w142:u8)  [unwired: 1 in]
          n45 = property class="DigNum (strict)"(reference=w150) -> (reference out=w149:refnum<vi>, error out=w151:errorcluster, "Value"=w136:u8)  [unwired: 1 in]
          n46 = property class="DigNum (strict)"(reference=w147) -> (reference out=w148:refnum<vi>, error out=w146:errorcluster, "Value"=w137:u8)  [unwired: 1 in]
          n47 = property class="DigNum (strict)"(reference=w127) -> (reference out=w126:refnum<vi>, error out=w128:errorcluster, "Value"=w131:u8)  [unwired: 1 in]
          n48 = property class="DigNum (strict)"(reference=w84) -> (reference out=w83:refnum<vi>, error out=w85:errorcluster, "Value"=w88:u8)  [unwired: 1 in]
          n49 = property class="DigNum (strict)"(reference=w79) -> (reference out=w78:refnum<vi>, error out=w80:errorcluster, "Value"=w68:u8)  [unwired: 1 in]
          n50 = property class="DigNum (strict)"(reference=w76) -> (reference out=w77:refnum<vi>, error out=w75:errorcluster, "Value"=w65:u8)  [unwired: 1 in]
          n51 = property class="DigNum (strict)"(reference=w73) -> (reference out=w72:refnum<vi>, error out=w74:errorcluster, "Value"=w59:u8)  [unwired: 1 in]
          n52 = property class="DigNum (strict)"(reference=w70) -> (reference out=w71:refnum<vi>, error out=w69:errorcluster, "Value"=w60:u8)  [unwired: 1 in]
          n53 = property class="DigNum (strict)"(reference=w54) -> (reference out=w53:refnum<vi>, error out=w55:errorcluster, "Value"=w58:u8)  [unwired: 1 in]
          n54 = property class="DigNum (strict)"(reference=w51) -> (reference out=w52:refnum<vi>, error out=w50:errorcluster, "Value"=w47:u8)  [unwired: 1 in]
          n55 = property class="DigNum (strict)"(reference=w42) -> (reference out=w41:refnum<vi>, error out=w43:errorcluster, "Value"=w46:u8)  [unwired: 1 in]
          n56 = Unbundle By Name(w40) -> ("Traction.Sequence ID"=w188:refnum<vi>)
          n57 = Increment(x=w185) -> (x+1=w184:u16)
          n58 = property class="DigNum (strict)"(reference=w188, "Value"=w184) -> (reference out=w186:refnum<vi>, error out=w187:errorcluster)  [unwired: 1 in]
          n59 = Close Reference(reference=w108, error in (no error)=w110) -> ()  [unwired: 1 out]
          n60 = Close Reference(reference=w107, error in (no error)=w105) -> ()  [unwired: 1 out]
          n61 = Close Reference(reference=w102, error in (no error)=w104) -> ()  [unwired: 1 out]
          n62 = Close Reference(reference=w101, error in (no error)=w99) -> ()  [unwired: 1 out]
          n63 = Close Reference(reference=w179, error in (no error)=w181) -> ()  [unwired: 1 out]
          n64 = Close Reference(reference=w177, error in (no error)=w175) -> ()  [unwired: 1 out]
          n65 = Close Reference(reference=w170, error in (no error)=w168) -> ()  [unwired: 1 out]
          n66 = Close Reference(reference=w114, error in (no error)=w116) -> ()  [unwired: 1 out]
          n67 = Close Reference(reference=w155, error in (no error)=w157) -> ()  [unwired: 1 out]
          n68 = Close Reference(reference=w154, error in (no error)=w152) -> ()  [unwired: 1 out]
          n69 = Close Reference(reference=w149, error in (no error)=w151) -> ()  [unwired: 1 out]
          n70 = Close Reference(reference=w148, error in (no error)=w146) -> ()  [unwired: 1 out]
          n71 = Close Reference(reference=w126, error in (no error)=w128) -> ()  [unwired: 1 out]
          n72 = Close Reference(reference=w83, error in (no error)=w85) -> ()  [unwired: 1 out]
          n73 = Close Reference(reference=w78, error in (no error)=w80) -> ()  [unwired: 1 out]
          n74 = Close Reference(reference=w77, error in (no error)=w75) -> ()  [unwired: 1 out]
          n75 = Close Reference(reference=w72, error in (no error)=w74) -> ()  [unwired: 1 out]
          n76 = Close Reference(reference=w71, error in (no error)=w69) -> ()  [unwired: 1 out]
          n77 = Close Reference(reference=w53, error in (no error)=w55) -> ()  [unwired: 1 out]
          n78 = Close Reference(reference=w52, error in (no error)=w50) -> ()  [unwired: 1 out]
          n79 = Close Reference(reference=w41, error in (no error)=w43) -> ()  [unwired: 1 out]
          n80 = Split Number(x=w184) -> (hi(x)=w183:u8, lo(x)=w182:u8)
          n81 = Type Cast(type=u8[] [], x=w165) -> (*(type *) &x=w167:u8[])
          n82 = Type Cast(type=u8[] [], x=w98) -> (*(type *) &x=w112:u8[])
          n83 = Type Cast(type=u8[] [], x=w95) -> (*(type *) &x=w96:u8[])
          n84 = Type Cast(type=u8[] [], x=w89) -> (*(type *) &x=w91:u8[])
          n85 = Type Cast(type=u8[] [], x=w90) -> (*(type *) &x=w94:u8[])
          n86 = Type Cast(type=u8[] [], x=w174) -> (*(type *) &x=w172:u8[])
          n87 = Type Cast(type=u8[] [], x=w119) -> (*(type *) &x=w117:u8[])
          n88 = Type Cast(type=u8[] [], x=w145) -> (*(type *) &x=w159:u8[])
          n89 = Type Cast(type=u8[] [], x=w142) -> (*(type *) &x=w143:u8[])
          n90 = Type Cast(type=u8[] [], x=w136) -> (*(type *) &x=w138:u8[])
          n91 = Type Cast(type=u8[] [], x=w137) -> (*(type *) &x=w141:u8[])
          n92 = Type Cast(type=u8[] [], x=w131) -> (*(type *) &x=w129:u8[])
          n93 = Type Cast(type=u8[] [], x=w88) -> (*(type *) &x=w86:u8[])
          n94 = Type Cast(type=u8[] [], x=w68) -> (*(type *) &x=w82:u8[])
          n95 = Type Cast(type=u8[] [], x=w65) -> (*(type *) &x=w66:u8[])
          n96 = Type Cast(type=u8[] [], x=w59) -> (*(type *) &x=w61:u8[])
          n97 = Type Cast(type=u8[] [], x=w60) -> (*(type *) &x=w64:u8[])
          n98 = Type Cast(type=u8[] [], x=w58) -> (*(type *) &x=w56:u8[])
          n99 = Type Cast(type=u8[] [], x=w47) -> (*(type *) &x=w49:u8[])
          n100 = Type Cast(type=u8[] [], x=w46) -> (*(type *) &x=w44:u8[])
          n101 = Close Reference(reference=w186, error in (no error)=w187) -> ()  [unwired: 1 out]
          n102 = Reverse 1D Array(array=w112) -> (reversed array=w39:u8[])
          n103 = Reverse 1D Array(array=w96) -> (reversed array=w38:u8[])
          n104 = Reverse 1D Array(array=w91) -> (reversed array=w37:u8[])
          n105 = Reverse 1D Array(array=w94) -> (reversed array=w36:u8[])
          n106 = Reverse 1D Array(array=w172) -> (reversed array=w173:u8[])
          n107 = Reverse 1D Array(array=w167) -> (reversed array=w164:u8[])
          n108 = Reverse 1D Array(array=w117) -> (reversed array=w113:u8[])
          n109 = Reverse 1D Array(array=w159) -> (reversed array=w120:u8[])
          n110 = Reverse 1D Array(array=w143) -> (reversed array=w121:u8[])
          n111 = Reverse 1D Array(array=w138) -> (reversed array=w122:u8[])
          n112 = Reverse 1D Array(array=w141) -> (reversed array=w123:u8[])
          n113 = Reverse 1D Array(array=w129) -> (reversed array=w124:u8[])
          n114 = Reverse 1D Array(array=w86) -> (reversed array=w35:u8[])
          n115 = Reverse 1D Array(array=w82) -> (reversed array=w34:u8[])
          n116 = Reverse 1D Array(array=w66) -> (reversed array=w33:u8[])
          n117 = Reverse 1D Array(array=w61) -> (reversed array=w32:u8[])
          n118 = Reverse 1D Array(array=w64) -> (reversed array=w31:u8[])
          n119 = Reverse 1D Array(array=w56) -> (reversed array=w30:u8[])
          n120 = Reverse 1D Array(array=w49) -> (reversed array=w29:u8[])
          n121 = Reverse 1D Array(array=w44) -> (reversed array=w28:u8[])
          n122 = Build Array (concatenate)(w182, w183, w178, w173, w164, w113, w120, w121, w122, w123, w124, w39, w38, w37, w36, w35, w34, w33, w32, w31, w30, w29, w28) -> (w163:u8[])
          n123 = String To IP(1:"192.168.1.8" ("name")) -> (0:w192:u32)
          n124 = Byte Array To String(unsigned byte array=w163) -> (string=w132:string)
          n125 = UDP Write(address=w192, port or service name=w193, connection ID=w160, data in=w132, 8:w191, 9:1 ("timeout ms (25000)")) -> (error out=w162:errorcluster, 3:w190:refnum<k16>)
          n126 = Unbundle By Name(w40) -> ("Traction.TRACTION WRITE"=w135:refnum<vi>)
          n127 = case shown="No Error" w162 {
            selector: w162 -> [w199 _]
            tunnel: w40 -> [w194 _]
            tunnel: [w199 _] -> w161
            frame No Error {
              n128 = Unbundle By Name(w194) -> ("Traction.Read TRACTION Temp"=w198:refnum<vi>)
              n129 = property class="Bool (strict)"(reference=w198, "Value"=TRUE) -> (reference out=w196:refnum<vi>, error out=w197:errorcluster)  [unwired: 1 in]
              n130 = Close Reference(reference=w196, error in (no error)=w197) -> ()  [unwired: 1 out]
            }
            frame Error {
            }
          }
          n131 = property class="Str"(reference=w135, "Value"=w132) -> (reference out=w133:refnum<vi>, error out=w134:errorcluster)  [unwired: 1 in]
          n132 = Close Reference(reference=w133, error in (no error)=w134) -> ()  [unwired: 1 out]
        }
        frame "CLOSE" {
          n133 = UDP Close(connection ID=w202, 8:w203) -> (error out=w201:errorcluster)  [unwired: 1 out]
        }
        frame "REINIT" {
          n134 = UDP Close(connection ID=w211, 8:w212) -> (error out=w210:errorcluster)  [unwired: 1 out]
          n135 = call "Stall Data Flow.vim"("value in"=w210, "milliseconds to wait"=u32 100) -> ("value out"=w207:errorcluster)  [unwired: 1 out]
          n136 = UDP Open(8:w207, 9:1 ("timeout ms (25000)"), 11:u16 8888 ("port")) -> (port=w205:refnum<k16>, 0:w206:errorcluster)  [unwired: 2 in, 1 out]
        }
      }
      "connection ID" <- w4
    }
    frame Error {
    }
  }
  "error out" <- w1
